vi "Target2.vi"() -> ()   [LabVIEW 2025]
uses:
  <vilib>/Platform/TimedLoop/XDataNode/timing_clust.ctl
  <vilib>/Platform/TimedLoop/XDataNode/nitl_modes.ctl
  <vilib>/Platform/TimedLoop/XDataNode/wakeup.ctl
  <vilib>/rvi/Emulation/niFpgaSctlEmulationGetInTimedLoop.vi
  <vilib>/rvi/Emulation/niFpgaEmulationReportErrorSimple.vi
  <vilib>/rvi/Emulation/niFpgaGetClockAttributes.vi
  <vilib>/rvi/Emulation/niFpgaCriticalErrorInLSC.vi
  <vilib>/rvi/interface/RandomDataEmulation/nirviRandomDataMultiElementFPGAFIFO.vi
  <instcachedir>/0/nirviRandomDataMultiElementFPGAFIFO_BE2FF10D3D6E420AB0291A02835C249E.lvgen/nirviRandomDataMultiElementFPGAFIFO_BE2FF10D3D6E420AB0291A02835C249E_001.vi
  <vilib>/rvi/interface/RandomDataEmulation/niFpgaRandomDataHandleErrors.vi
  <vilib>/platform/TimedLoop/XDataNode/XDataNode.xnode
  <vilib>/rvi/DataTransferAndStorage/Container/XNode/niFpgaContainer.xnode
  <vilib>/rvi/interface/RandomDataEmulation/nirviRandomDataFpgaMultiElementTemplate.vi
  <vilib>/Platform/TimedLoop/XDataNode/XDNodeRunTimeDep.lvlib
panel:
  out "FIFO D.2":fxp<+,1,2>[](array[numeric])=[2.0, 2.0]
  out "FIFO D":fxp<+,1,2>[](array[numeric])=[2.0, 2.0]
  out "FIFO C":fxp<+,1,1>[](array[numeric])=[1.0, 1.0]
  out "FIFO C.2":fxp<+,1,1>[](array[numeric])=[1.0, 1.0]
  out "appended array":fxp<+/-,32,16>[](array[numeric])
  out "appended array 2":fxp<+/-,32,16>[](array[numeric])
  out "element":fxp<+/-,32,16>
  out "element 2":fxp<+/-,32,16>
  out "element 3":fxp<+/-,32,16>
  out "element 4":fxp<+/-,32,16>
  out "cr":fxp<+/-,32,16>[](array[numeric])
  out "Numeric":i32
  out "Case Number":i16
  out "interleaved array":fxp<+/-,32,16>[](array[numeric])
  out "interleaved array 2":fxp<+/-,32,16>[](array[numeric])
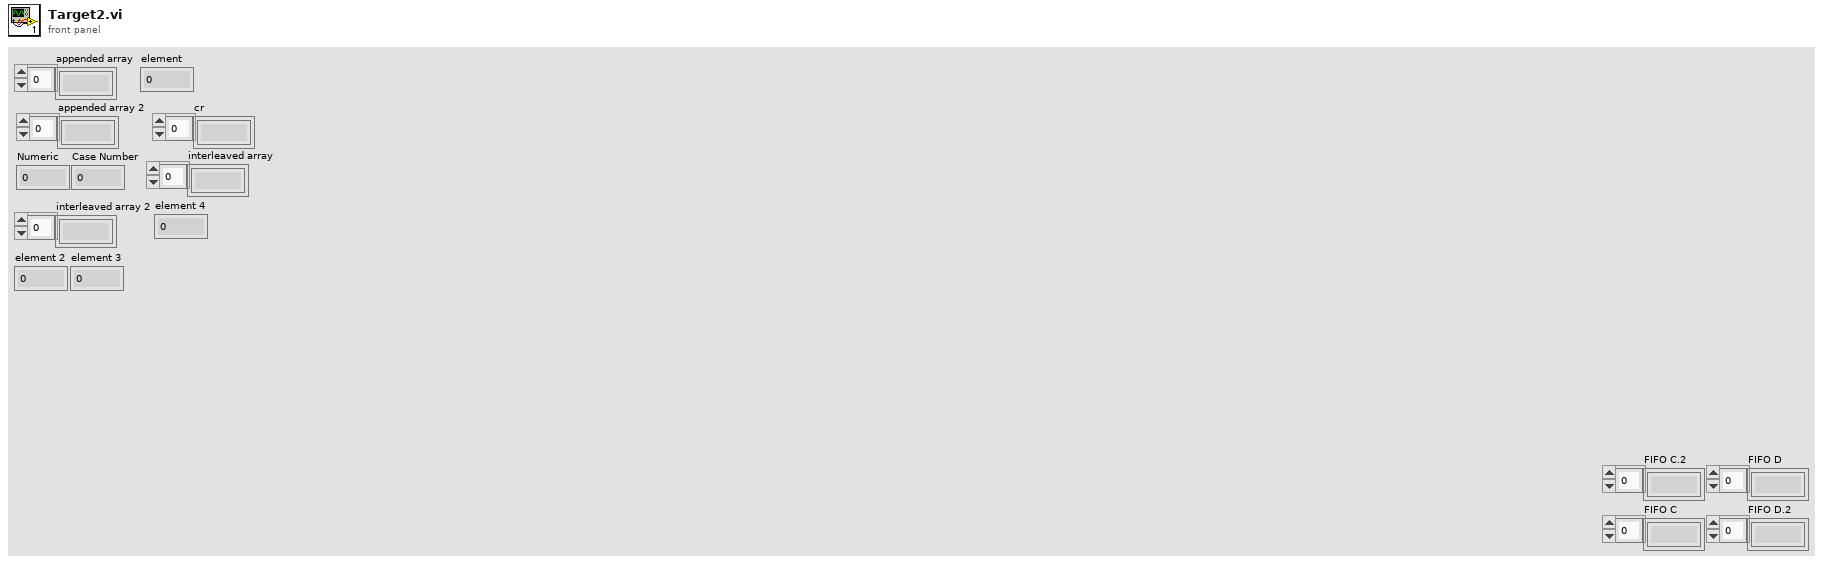
[diagram p1: front panel]
types:
  T1 = typedef "XDNodeRunTimeDep.lvlib/timing_clust.ctl" = cluster{"Expected End [f-1]":u64, "Actual End [f-1]":u64, "Finished Late? [f-1]":bool, "Expected End [i-1]":u64, "Actual End [i-1]":u64, "Finished Late? [i-1]":bool, "Expected Start [i]":u64, "Actual Start [i]":u64, "Expected Start [f]":u64, "Actual Start [f]":u64, "Source Name":string, "Structure Name":string, "Period":i64, "Deadline":i64, "Offset":i64, "Start":i64, "Priority":i32, "Timeout":i32, "Mode":T2, "Wakeup Reason":T3, "Error":errorcluster, "Source Type":string, "Secondary Source Type":string, "Global End Time":u64, "Global Start Time":u64, "Frame Duration":u64, "Iteration Duration":u64, "Assigned CPU":i32, "I/O Scan Engine Mode":u32}
  T2 = typedef "XDNodeRunTimeDep.lvlib/nitl_modes.ctl" = enum32{"No Change", "Process missed periods, maintain original phase", "Discard missed periods, maintain original phase", "Process missed periods, ignore original phase", "Discard missed periods, ignore original phase"}
  T3 = typedef "XDNodeRunTimeDep.lvlib/wakeup.ctl" = enum32{"Normal", "Aborted", "Asynchronous wakeup", "Timing source error", "Timed loop error", "Timeout"}
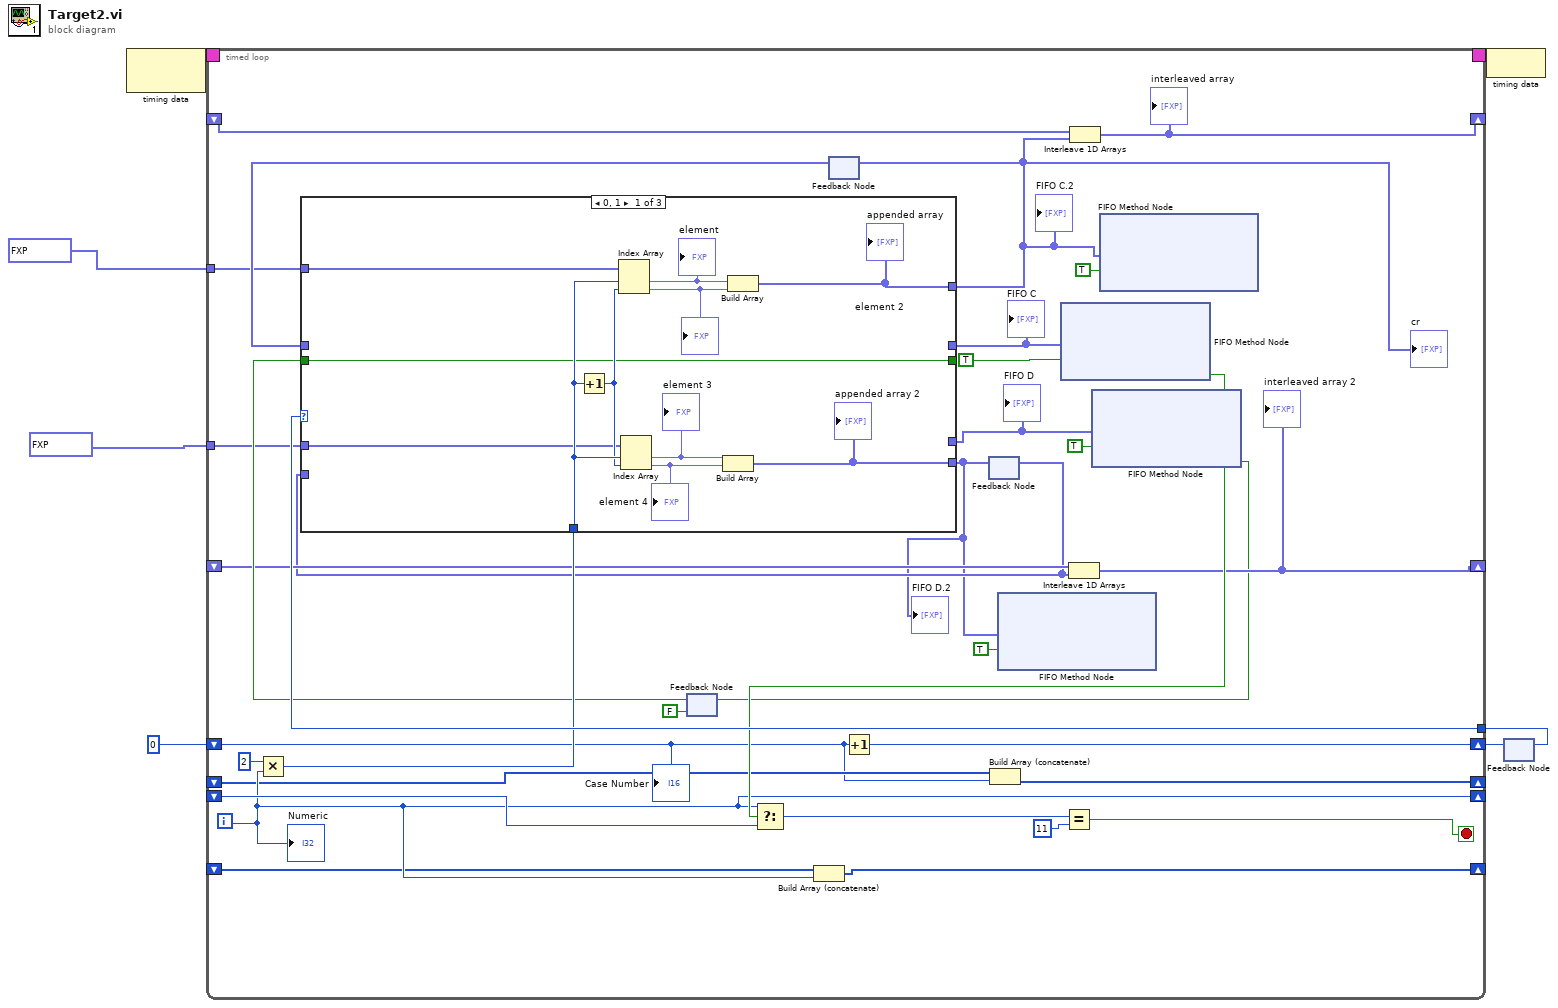
[diagram p0: block diagram]
diagram:
  n1 = node-c288() -> (w7:T1)  [unwired: 1 in]
  n2 = feedback #1() -> (w3:i16)  [unwired: 1 in]
  n3 = timed-loop {
    timing: w7 -> [_]
    timing-out: [_] -> w6
    shift-right: [w41] -> w4
    shift-left: i16 0 -> [w17]
    tunnel: w3 -> [w40]
    shift-right: [w22] -> _
    shift-left: _ -> [w36]
    tunnel: fxp<+,1,1>[] [1.0, 1.0] -> [w30]
    tunnel: fxp<+,1,2>[] [2.0, 2.0] -> [w29]
    shift-right: [w24] -> _
    shift-left: _ -> [w25]
    shift-right: [w23] -> _
    shift-left: _ -> [w26]
    shift-right: [w20] -> _
    shift-left: _ -> [w21]
    shift-right: [w18] -> _
    shift-left: _ -> [w19]
    i -> [w22]
    stop <- w33 stop-if-true
    n4 = Multiply(x=2, y=w22) -> (x*y=w38:i32)
    n5 = feedback #2(FALSE ("output valid")) -> (w32:bool)
    n6 = Build Array (concatenate)(w21, w22) -> (w20:i32[])
    n7 = feedback #3() -> (w37:fxp<+,1,1>[])  [unwired: 1 in]
    n8 = Increment(x=w17) -> (x+1=w41:i16)
    n9 = feedback #4() -> (w16:fxp<+,1,2>[])  [unwired: 1 in]
    n10 = case shown="0, 1" w40 {
      tunnel: [w48 _ _] -> w11
      tunnel: [w47 _ _] -> w8
      tunnel: w38 -> [w46 _ _]
      tunnel: w37 -> [_ _ w56]
      tunnel: w32 -> [w42 w53 w55]
      tunnel: w30 -> [w44 _ _]
      tunnel: w29 -> [w43 _ _]
      tunnel: [_ _ w56] -> w27
      tunnel: [w42 w53 w55] -> _
      tunnel: w16 -> [_ _ w54]
      tunnel: [_ _ w54] -> w15
      frame 0, 1 {
        n11 = Increment(x=w46) -> (x+1=w45:i32)
        n12 = Index Array(array=w44, index #1=w46, index #2=w45) -> (element #1=w50:fxp<+,1,1>, element #2=w49:fxp<+,1,1>)
        "element" <- w50
        "element 2" <- w49
        n13 = Index Array(array=w43, index #1=w46, index #2=w45) -> (element #1=w52:fxp<+,1,2>, element #2=w51:fxp<+,1,2>)
        "element 3" <- w52
        "element 4" <- w51
        n14 = Build Array(w52, w51) -> (w47:fxp<+,1,2>[])
        "appended array 2" <- w47
        n15 = Build Array(w50, w49) -> (w48:fxp<+,1,1>[])
        "appended array" <- w48
      }
      frame 3, Default {
      }
      frame 10, 11 {
      }
    }
    "cr" <- w11
    "FIFO C.2" <- w11
    "FIFO C" <- w27
    "FIFO D" <- w15
    "FIFO D.2" <- w8
    n16 = feedback-in #3(w11) -> ()
    n17 = feedback-in #4(w8) -> ()
    n18 = Build Array (concatenate)(w19, w17) -> (w18:i16[])
    n19 = xnode ("FIFO Method Node")("Element"=w8, "Input Valid"=TRUE) -> ()  [unwired: 1 in, 2 out]
    n20 = xnode ("FIFO Method Node")("Element"=w27, "Input Valid"=TRUE) -> ("Ready for Input"=w28:bool)  [unwired: 1 in, 1 out]
    n21 = Select(t=w22, s=w28, f=w36) -> (s? t:f=w35:i32)
    n22 = Equal?(x=w35, y=11) -> (x = y?=w33:bool)
    n23 = Interleave 1D Arrays(w26, w16) -> (w23:fxp<+,1,2>[])
    "interleaved array 2" <- w23
    n24 = Interleave 1D Arrays(w25, w11) -> (w24:fxp<+,1,1>[])
    "interleaved array" <- w24
    n25 = xnode ("FIFO Method Node")("Element"=w15, "Input Valid"=TRUE) -> ("Ready for Input"=w14:bool)  [unwired: 1 in, 1 out]
    n26 = feedback-in #2(w14) -> ()
    n27 = xnode ("FIFO Method Node")("Element"=w11, "Input Valid"=TRUE) -> ()  [unwired: 1 in, 2 out]
    "Numeric" <- w22
    "Case Number" <- w17
  }
  n28 = node-c288(w6) -> ()
  n29 = feedback-in #1(w4) -> ()
